vi "GPIBreceive.vi"(2 "timeout ms":u32=4294967295 format="%.0x", 3 "address string":string, 4 "byte count":i32, 7 "source":string, 8 "read mode":i32(ring) items=["terminate read on EOI or byte count", "terminate read on EOI, byte count, or CR", "terminate read on EOI, byte count, or LF"], 9 "error in":T1) -> (0 "read buffer":string, 5 "status":bool[](array[boolean]), 6 "error out":T1)   [LabVIEW 2013, in "InstrControl.lvclass"]
doc: "Sends a string to a message based instrument. You must supply the address string of the instrument. A byte count value is required in order to tell the VI how many bytes can be returned by the VI. Select the appropriate read mode to terminate the receive function correctly."
uses:
  InstrControl.lvclass
panel:
  in  "[empty array]":bool[](array[boolean])
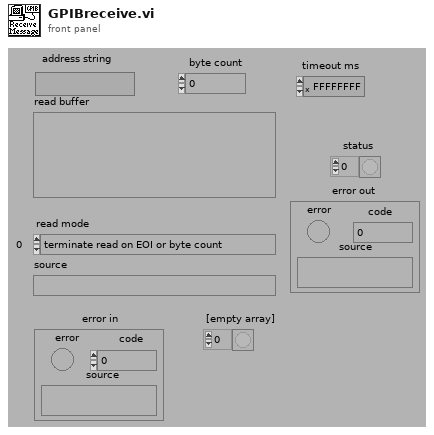
[diagram p1: front panel]
types:
  T1 = cluster{"error":bool, "code":i32, "source":string}
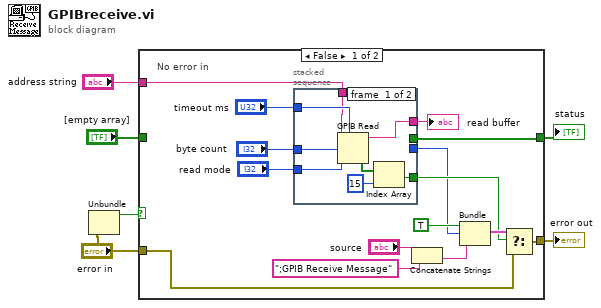
[diagram p0: block diagram]
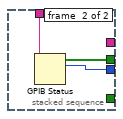
[diagram p2: hidden frame]
diagram:
  n1 = Unbundle("error in") -> ("error"=w2:bool)  [unwired: 2 out]
  n2 = case shown="False" w2 {
    tunnel: "[empty array]" -> [_ w33]
    tunnel: [w17 w33] -> w4
    tunnel: [w20 w34] -> w5
    tunnel: "error in" -> [w12 w34]
    tunnel: "address string" -> [w7 _]
    frame False {
      # "No error in"
      n3 = stacked-sequence {
        tunnel: [_ w32] -> w17
        tunnel: [w27 _] -> w18
        tunnel: [_ w31] -> w16
        tunnel: "timeout ms" -> [w26 _]
        tunnel: "read mode" -> [w25 _]
        tunnel: "byte count" -> [w24 _]
        tunnel: [w23 _] -> w8
        tunnel: w7 -> [w22 w30]
        frame #0 {
          n4 = GPIB Read(0:w22, 1:w24, 2:w25, 4:w26) -> (5:w23:string, 6:w28:bool[])  [unwired: 1 in, 1 out]
          n5 = Index Array(array=w28, index=15) -> (element=w27:bool)
        }
        frame #1 {
          n6 = GPIB Status(0:w30) -> (2:w32:bool[], 3:w31:i16)  [unwired: 1 in, 2 out]
        }
      }
      "read buffer" <- w8
      n7 = Concatenate Strings("source", ";GPIB Receive Message") -> (w13:string)
      n8 = Bundle(TRUE, "GPIB error"=w16, w13) -> (w21:cluster{bool, "GPIB error":i16, string})  [unwired: 1 in]
      n9 = Select(t=w21, s=w18, f=w12) -> (s? t:f=w20:T1)
    }
    frame True {
      # "Error in"
    }
  }
  "status" <- w4
  "error out" <- w5
